vi "Top Level.vi"() -> ()   [LabVIEW 2013]
uses:
  Classes/OSSP_Problem.lvclass
  Classes/SA.lvclass
  Classes/SA_Class/Controls/Solution_SA.ctl
  GA/Controls/Scheduler Type.ctl
  Controls/States_SA.ctl
  Classes/SA.lvclass/SA.ctl
  Classes/GanntChart_Class/Operation to Machine Job Tuple.vi
  Classes/GanntChart_Class/Check Other Machines for Schedule Time.vi
  Classes/GanntChart_Class/Schedule Job.vi
  Classes/GanntChart_Class/Find Gaps on Particular Machine.vi
  Classes/GanntChart_Class/Increment Number of Jobs on Machine.vi
  Classes/GanntChart_Class/Find Job On Other Machines.vi
  Classes/GanntChart.lvclass
panel:
  out "Thermometer":dbl(slide) scale=0.0..1000.0
  in  "Scheduler":T1
  out "Final Solution":T2
  out "SA.lvclass":refnum<class "SA.lvclass">
  out "OSSP_Problem.lvclass":refnum<class "OSSP_Problem.lvclass">
  in  "Stop Temperature":dbl=1.0 format="%#_13g"
  in  "Cooling Rate":dbl=0.003
  in  "Starting Temperature":dbl=10000.0
  out "error out":errorcluster
  in  "error in (no error)":errorcluster
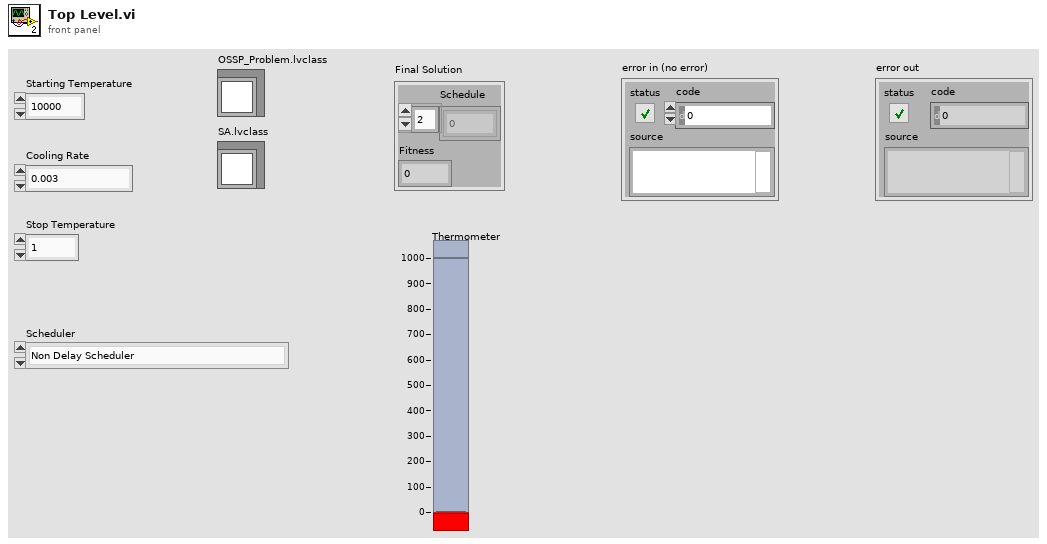
[diagram p1: front panel]
types:
  T1 = typedef "Scheduler Type.ctl" = enum16{"Non Delay Scheduler", "My Scheduler"}
  T2 = typedef "Solution_SA.ctl" = cluster{"Schedule":u16[], "Fitness":u16}
  T3 = typedef "States_SA.ctl" = enum16{"Init", "Read Problem", "Sort Problem", "Generate and Evaluate Current Solution", "Perturb Cur Solution and Eval New Solution", "Make Decision", "Keep Track of Best Solution", "Cool", "Output Final Solution", "Stop"}
  T4 = typedef "GanntChart_Element.ctl" = cluster{"Operation Number":i32, "Job Number":i32, "Start Time":i32, "Procesing Time":u16, "End Time":i32}
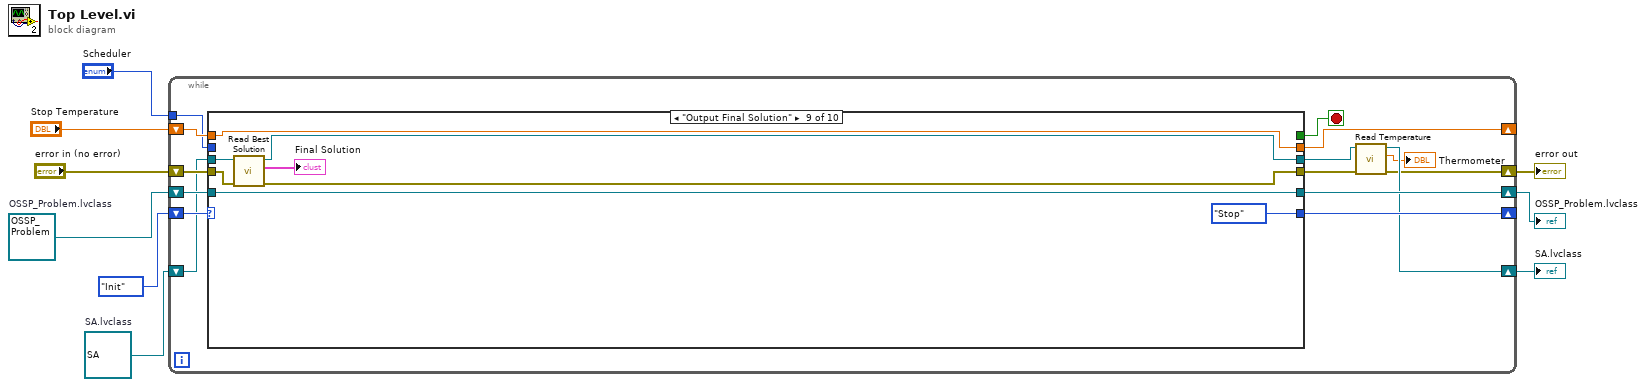
[diagram p0: block diagram]
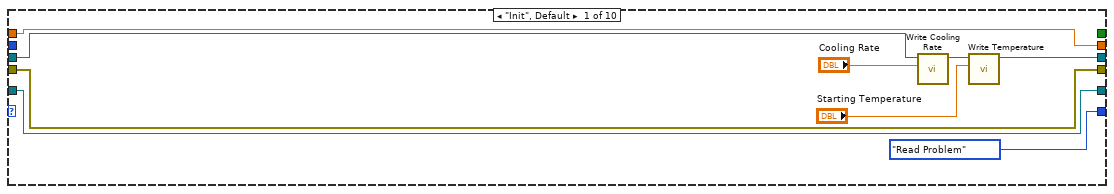
[diagram p2: hidden frame]
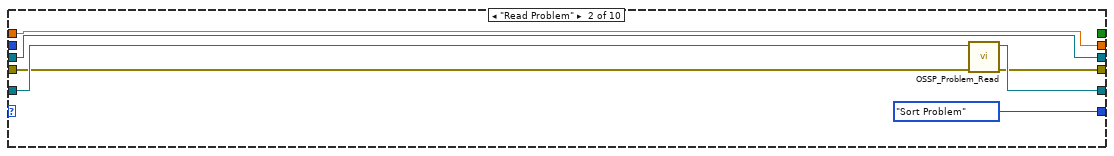
[diagram p3: hidden frame]
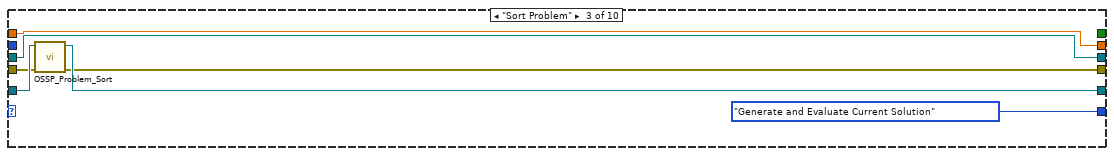
[diagram p4: hidden frame]
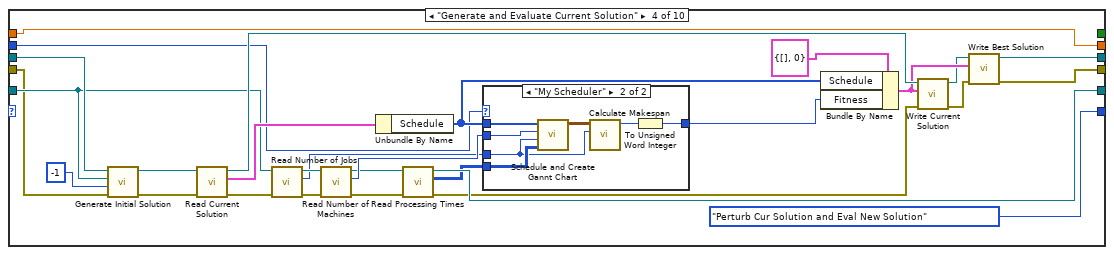
[diagram p5: hidden frame]
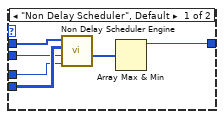
[diagram p6: hidden frame]
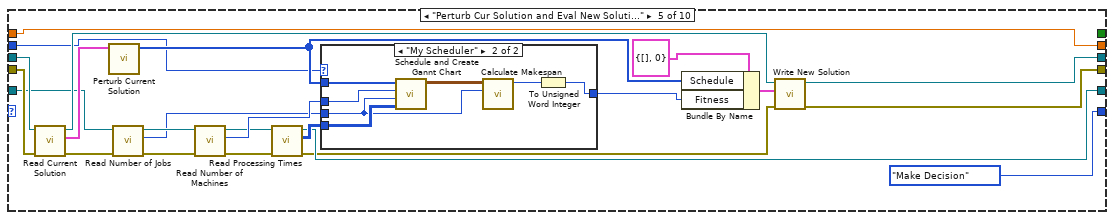
[diagram p7: hidden frame]
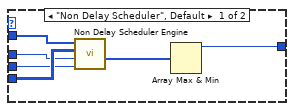
[diagram p8: hidden frame]
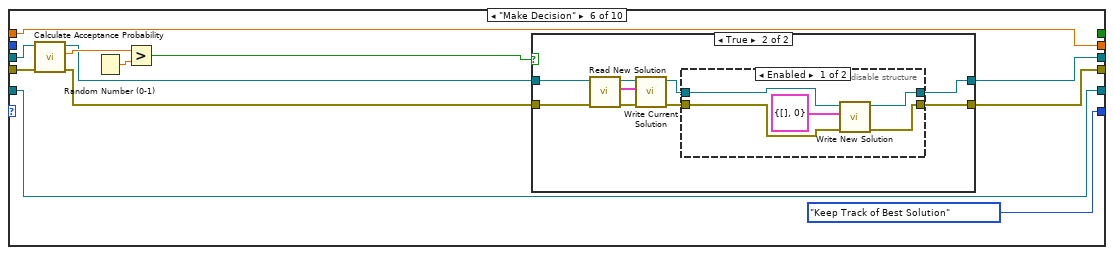
[diagram p9: hidden frame]
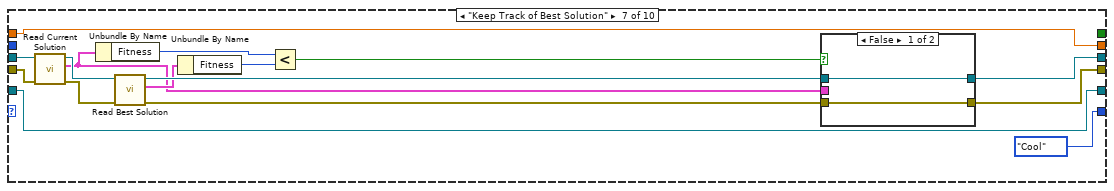
[diagram p12: hidden frame]
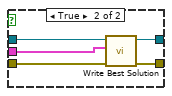
[diagram p13: hidden frame]
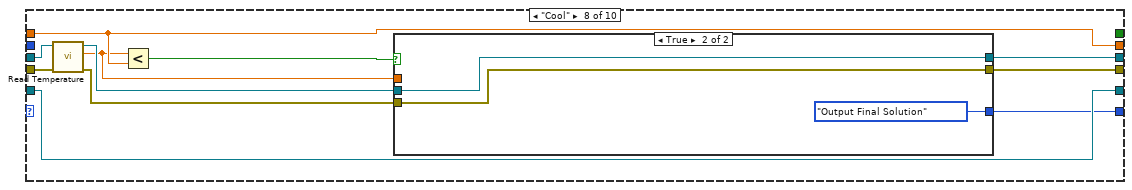
[diagram p14: hidden frame]
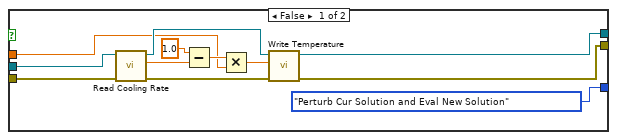
[diagram p15: hidden frame]
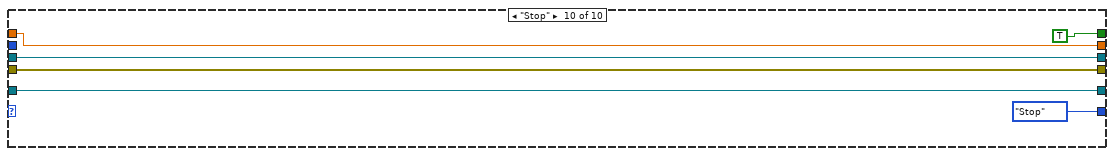
[diagram p16: hidden frame]
diagram:
  w5 = refnum<class "SA.lvclass"> refnum  # SA.lvclass
  w8 = refnum<class "OSSP_Problem.lvclass"> refnum  # OSSP_Problem.lvclass
  n1 = while {
    shift-right: [w23] -> _
    shift-left: States_SA."Init" -> [w24]
    shift-right: [w19] -> w3
    shift-left: w8 -> [w21]
    shift-right: [w10] -> w6
    shift-left: "error in (no error)" -> [w20]
    shift-right: [w13] -> w2
    shift-left: w5 -> [w18]
    shift-right: [w17] -> _
    shift-left: "Stop Temperature" -> [w16]
    tunnel: "Scheduler" -> [w15]
    stop <- w22 stop-if-true
    n2 = case shown="\"Output Final Solution\"" w24 {
      tunnel: [States_SA."Read Problem" States_SA."Sort Problem" States_SA."Generate and Evaluate Current Solution" States_SA."Perturb Cur Solution and Eval New Solution" States_SA."Make Decision" States_SA."Keep Track of Best Solution" States_SA."Cool" w187 States_SA."Stop" States_SA."Stop"] -> w23
      tunnel: [_ _ _ _ _ _ _ _ _ TRUE] -> w22
      tunnel: w21 -> [w32 w39 w46 w69 w101 w138 w172 w190 w213 w217]
      tunnel: [w31 w36 w43 w50 w105 w133 w167 w184 w208 w216] -> w11
      tunnel: w20 -> [w31 w37 w44 w67 w111 w135 w170 w188 w209 w216]
      tunnel: [w32 w38 w45 w72 w93 w138 w172 w190 w213 w217] -> w19
      tunnel: w18 -> [w27 w35 w42 w70 w108 w134 w169 w189 w211 w215]
      tunnel: [w26 w35 w42 w52 w107 w132 w168 w182 w210 w215] -> w14
      tunnel: [w25 w34 w41 w76 w113 w137 w171 w181 w212 w214] -> w17
      tunnel: w16 -> [w25 w34 w41 w76 w113 w137 w171 w181 w212 w214]
      tunnel: w15 -> [_ _ _ w48 w91 _ _ _ _ _]
      frame "Init", Default {
        n3 = call "Write Cooling Rate.vi"("Cooling Rate"="Cooling Rate", "SA in"=w27) -> ("SA out"=w29:refnum<class "SA.lvclass">)  [unwired: 8 in, 1 out]
        n4 = call "Write Temperature.vi"("Temperature"="Starting Temperature", "SA in"=w29) -> ("SA out"=w26:refnum<class "SA.lvclass">)  [unwired: 8 in, 1 out]
      }
      frame "Read Problem" {
        n5 = call "OSSP_Problem_Read.vi"("error in (no error)"=w37, "OSSP_Problem.lvclass In"=w39) -> ("error out"=w36:errorcluster, "OSSP_Problem.lvclass Out"=w38:refnum<class "OSSP_Problem.lvclass">)  [unwired: 8 in]
      }
      frame "Sort Problem" {
        n6 = call "OSSP_Problem_Sort.vi"("error in (no error)"=w44, "OSSP_Problem.lvclass In"=w46) -> ("error out"=w43:errorcluster, "OSSP_Problem.lvclass Out"=w45:refnum<class "OSSP_Problem.lvclass">)  [unwired: 8 in]
      }
      frame "Generate and Evaluate Current Solution" {
        n7 = call "Generate Initial Solution.vi"("error in (no error)"=w67, "seed"=-1, "OSSP_Problem In"=w69, "SA in"=w70) -> ("error out"=w66:errorcluster, "SA out"=w65:refnum<class "SA.lvclass">)  [unwired: 6 in]
        n8 = call "Read Current Solution.vi"("error in (no error)"=w66, "SA in"=w65) -> ("error out"=w73:errorcluster, "Solution"=w74:T2, "SA out"=w71:refnum<class "SA.lvclass">)  [unwired: 7 in]
        n9 = call-dynamic "Read Number of Jobs.vi"("error in (no error)"=w73, "OSSP_Problem in"=w69) -> ("error out"=w62:errorcluster, "Number of Jobs"=w58:i32, "OSSP_Problem out"=w63:refnum<class "OSSP_Problem.lvclass">)  [unwired: 7 in]
        n10 = call-dynamic "Read Number of Machines.vi"("error in (no error)"=w62, "OSSP_Problem in"=w63) -> ("error out"=w61:errorcluster, "Number of Machines"=w64:i32, "OSSP_Problem out"=w60:refnum<class "OSSP_Problem.lvclass">)  [unwired: 7 in]
        n11 = Unbundle By Name(w74) -> ("Schedule"=w55:u16[])
        n12 = call-dynamic "Read Processing Times.vi"("error in (no error)"=w61, "OSSP_Problem in"=w60) -> ("error out"=w56:errorcluster, "Processing Times"=w59:u16[][], "OSSP_Problem out"=w72:refnum<class "OSSP_Problem.lvclass">)  [unwired: 7 in]
        n13 = case shown="\"My Scheduler\"" w48 {
          tunnel: w64 -> [w80 w89]
          tunnel: w59 -> [w81 w88]
          tunnel: w58 -> [w79 w86]
          tunnel: [w77 w83] -> w49
          tunnel: w55 -> [w82 w85]
          frame "Non Delay Scheduler", Default {
            n14 = call "Non Delay Scheduler Engine.vi"("Number of  Jobs"=w79, "Number of Machines"=w80, "Processing Times"=w81, "Schedule"=w82) -> ("Job Completion Times"=w78:u16[])  [unwired: 3 in, 4 out]
            n15 = Array Max & Min(array=w78) -> (max value=w77:u16)  [unwired: 3 out]
          }
          frame "My Scheduler" {
            n16 = call "Schedule and Create Gannt Chart.vi"("Processing Times (Rows Mach.Cols Jobs)"=w88, "Number of Jobs"=w86, "Number of Machines"=w89, "Schedule"=w85) -> ("Gannt Chart Out"=w87:T4[][])  [unwired: 6 in, 1 out]
            n17 = call "Calculate Makespan.vi"("Number of Jobs"=w86, "Gannt Chart In"=w87) -> ("Makespan"=w84:i32)  [unwired: 9 in]
            n18 = To Unsigned Word Integer(number=w84) -> (unsigned 16bit integer=w83:u16)
          }
        }
        n19 = Bundle By Name(cluster=T2 {"Schedule"=[], "Fitness"=0} ("Solution"), "Schedule"=w55, "Fitness"=w49) -> (w54:T2)
        n20 = call "Write Current Solution.vi"("error in (no error)"=w56, "Solution"=w54, "SA in"=w71) -> ("error out"=w51:errorcluster, "SA out"=w53:refnum<class "SA.lvclass">)  [unwired: 7 in]
        n21 = call "Write Best Solution.vi"("error in (no error)"=w51, "Solution"=w54, "SA in"=w53) -> ("error out"=w50:errorcluster, "SA out"=w52:refnum<class "SA.lvclass">)  [unwired: 7 in]
      }
      frame "Perturb Cur Solution and Eval New Solution" {
        n22 = call "Read Current Solution.vi"("error in (no error)"=w111, "SA in"=w108) -> ("error out"=w102:errorcluster, "Solution"=w106:T2, "SA out"=w103:refnum<class "SA.lvclass">)  [unwired: 7 in]
        n23 = call "Perturb Current Solution.vi"("Solution"=w106) -> ("Schedule"=w104:u16[])  [unwired: 10 in]
        n24 = call-dynamic "Read Number of Jobs.vi"("error in (no error)"=w102, "OSSP_Problem in"=w101) -> ("error out"=w98:errorcluster, "Number of Jobs"=w94:i32, "OSSP_Problem out"=w99:refnum<class "OSSP_Problem.lvclass">)  [unwired: 7 in]
        n25 = call-dynamic "Read Number of Machines.vi"("error in (no error)"=w98, "OSSP_Problem in"=w99) -> ("error out"=w97:errorcluster, "Number of Machines"=w100:i32, "OSSP_Problem out"=w96:refnum<class "OSSP_Problem.lvclass">)  [unwired: 7 in]
        n26 = call-dynamic "Read Processing Times.vi"("error in (no error)"=w97, "OSSP_Problem in"=w96) -> ("error out"=w92:errorcluster, "Processing Times"=w95:u16[][], "OSSP_Problem out"=w93:refnum<class "OSSP_Problem.lvclass">)  [unwired: 7 in]
        n27 = case shown="\"My Scheduler\"" w91 {
          tunnel: w104 -> [w119 w126]
          tunnel: w100 -> [w116 w125]
          tunnel: w95 -> [w118 w124]
          tunnel: w94 -> [w117 w122]
          tunnel: [w114 w120] -> w90
          frame "Non Delay Scheduler", Default {
            n28 = call "Non Delay Scheduler Engine.vi"("Number of  Jobs"=w117, "Number of Machines"=w116, "Processing Times"=w118, "Schedule"=w119) -> ("Job Completion Times"=w115:u16[])  [unwired: 3 in, 4 out]
            n29 = Array Max & Min(array=w115) -> (max value=w114:u16)  [unwired: 3 out]
          }
          frame "My Scheduler" {
            n30 = call "Schedule and Create Gannt Chart.vi"("Processing Times (Rows Mach.Cols Jobs)"=w124, "Number of Jobs"=w122, "Number of Machines"=w125, "Schedule"=w126) -> ("Gannt Chart Out"=w123:T4[][])  [unwired: 6 in, 1 out]
            n31 = call "Calculate Makespan.vi"("Number of Jobs"=w122, "Gannt Chart In"=w123) -> ("Makespan"=w121:i32)  [unwired: 9 in]
            n32 = To Unsigned Word Integer(number=w121) -> (unsigned 16bit integer=w120:u16)
          }
        }
        n33 = Bundle By Name(cluster=T2 {"Schedule"=[], "Fitness"=0} ("Solution"), "Schedule"=w104, "Fitness"=w90) -> (w109:T2)
        n34 = call "Write New Solution.vi"("error in (no error)"=w92, "Solution"=w109, "SA in"=w103) -> ("error out"=w105:errorcluster, "SA out"=w107:refnum<class "SA.lvclass">)  [unwired: 7 in]
      }
      frame "Make Decision" {
        n35 = call "Calculate Acceptance Probability.vi"("error in (no error)"=w135, "SA in"=w134) -> ("error out"=w128:errorcluster, "Acceptance Probability"=w131:dbl, "SA out"=w127:refnum<class "SA.lvclass">)  [unwired: 7 in]
        n36 = Random Number (0-1)() -> (number: 0 to 1=w130:dbl)
        n37 = Greater?(x=w131, y=w130) -> (0:w129:bool)
        n38 = case shown="True" w129 {
          tunnel: w127 -> [w139 w149]
          tunnel: w128 -> [w140 w148]
          tunnel: [w140 w141] -> w133
          tunnel: [w139 w142] -> w132
          frame False {
          }
          frame True {
            n39 = call "Read New Solution.vi"("error in (no error)"=w148, "SA in"=w149) -> ("error out"=w147:errorcluster, "Solution"=w145:T2, "SA out"=w146:refnum<class "SA.lvclass">)  [unwired: 7 in]
            n40 = call "Write Current Solution.vi"("error in (no error)"=w147, "Solution"=w145, "SA in"=w146) -> ("error out"=w143:errorcluster, "SA out"=w144:refnum<class "SA.lvclass">)  [unwired: 7 in]
            n41 = disable-structure shown="Enabled" {
              disable-tunnel: w144 -> [w154 w156]
              disable-tunnel: w143 -> [w153 w155]
              disable-tunnel: [w152 w156] -> w142
              disable-tunnel: [w151 w155] -> w141
              frame Enabled {
                n42 = call "Write New Solution.vi"("error in (no error)"=w153, "Solution"=T2 {"Schedule"=[], "Fitness"=0}, "SA in"=w154) -> ("error out"=w151:errorcluster, "SA out"=w152:refnum<class "SA.lvclass">)  [unwired: 7 in]
              }
              frame Disabled {
              }
            }
          }
        }
      }
      frame "Keep Track of Best Solution" {
        n43 = call "Read Current Solution.vi"("error in (no error)"=w170, "SA in"=w169) -> ("error out"=w162:errorcluster, "Solution"=w157:T2, "SA out"=w165:refnum<class "SA.lvclass">)  [unwired: 7 in]
        n44 = Unbundle By Name(w157) -> ("Fitness"=w161:u16)
        n45 = call "Read Best Solution.vi"("error in (no error)"=w162, "SA in"=w165) -> ("error out"=w163:errorcluster, "Solution"=w160:T2, "SA out"=w164:refnum<class "SA.lvclass">)  [unwired: 7 in]
        n46 = Unbundle By Name(w160) -> ("Fitness"=w159:u16)
        n47 = Less?(x=w161, y=w159) -> (x < y?=w158:bool)
        n48 = case shown="False" w158 {
          tunnel: w164 -> [w174 w179]
          tunnel: [w174 w178] -> w168
          tunnel: w163 -> [w173 w177]
          tunnel: [w173 w176] -> w167
          tunnel: w157 -> [_ w175]
          frame False {
          }
          frame True {
            n49 = call "Write Best Solution.vi"("error in (no error)"=w177, "Solution"=w175, "SA in"=w179) -> ("error out"=w176:errorcluster, "SA out"=w178:refnum<class "SA.lvclass">)  [unwired: 7 in]
          }
        }
      }
      frame "Cool" {
        n50 = call "Read Temperature.vi"("error in (no error)"=w188, "SA in"=w189) -> ("error out"=w185:errorcluster, "Temperature"=w180:dbl, "SA out"=w183:refnum<class "SA.lvclass">)  [unwired: 7 in]
        n51 = Less?(x=w180, y=w181) -> (x < y?=w186:bool)
        n52 = case shown="True" w186 {
          tunnel: [States_SA."Perturb Cur Solution and Eval New Solution" ("f") States_SA."Output Final Solution"] -> w187
          tunnel: w183 -> [w199 w204]
          tunnel: w185 -> [w197 w203]
          tunnel: [w201 w203] -> w184
          tunnel: [w200 w204] -> w182
          tunnel: w180 -> [w191 _]
          frame False {
            n53 = call "Read Cooling Rate.vi"("error in (no error)"=w197, "SA in"=w199) -> ("error out"=w196:errorcluster, "Cooling Rate"=w194:dbl, "SA out"=w198:refnum<class "SA.lvclass">)  [unwired: 7 in]
            n54 = Subtract(x=1.0, y=w194) -> (x-y=w193:dbl)
            n55 = Multiply(x=w193, y=w191) -> (x*y=w192:dbl)
            n56 = call "Write Temperature.vi"("error in (no error)"=w196, "Temperature"=w192, "SA in"=w198) -> ("error out"=w201:errorcluster, "SA out"=w200:refnum<class "SA.lvclass">)  [unwired: 7 in]
          }
          frame True {
          }
        }
      }
      frame "Output Final Solution" {
        n57 = call "Read Best Solution.vi"("error in (no error)"=w209, "SA in"=w211) -> ("error out"=w208:errorcluster, "Solution"=→"Final Solution":T2, "SA out"=w210:refnum<class "SA.lvclass">)  [unwired: 7 in]
      }
      frame "Stop" {
      }
    }
    n58 = call "Read Temperature.vi"("error in (no error)"=w11, "SA in"=w14) -> ("error out"=w10:errorcluster, "Temperature"=→"Thermometer":dbl, "SA out"=w13:refnum<class "SA.lvclass">)  [unwired: 7 in]
  }
  "error out" <- w6
  "OSSP_Problem.lvclass" <- w3
  "SA.lvclass" <- w2
